vi "Initialize.vi"(8 "error in (no error)":errorcluster, 10 "DeviceName":string, 11 "MagSpec_Bella in":refnum<class "MagSpec_Bella.lvclass">) -> (0 "error out":errorcluster, 1 "new command(s)":string, 2 "DeviceName":string, 3 "MagSpec_Bella out":refnum<class "MagSpec_Bella.lvclass">)   [LabVIEW 2020, in "MagSpec_Bella.lvclass"]
uses:
  MagSpec_Bella.lvclass
  source/Device Drivers/BaseDriver/BaseDriver.lvclass
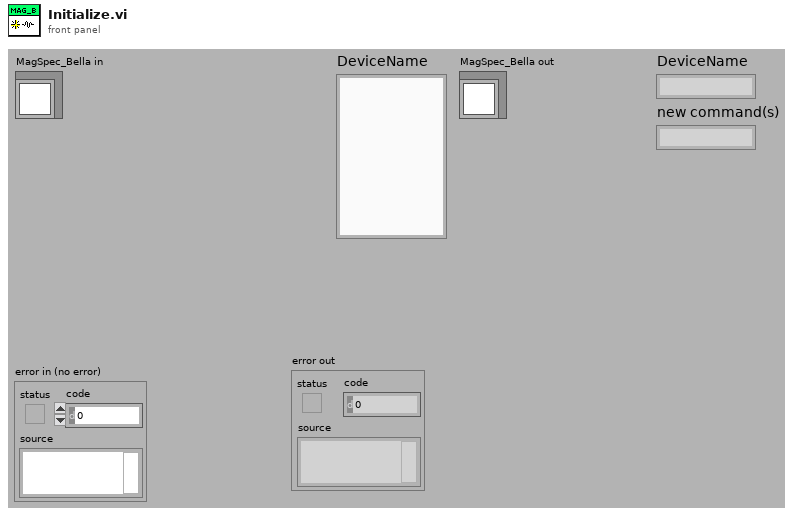
[diagram p1: front panel]
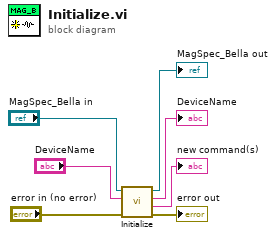
[diagram p0: block diagram]
diagram:
  n1 = call-parent "Initialize.vi"("error in (no error)"="error in (no error)", "DeviceName"="DeviceName", "BaseDriver in"="MagSpec_Bella in") -> ("error out"=→"error out":errorcluster, "new command(s)"=→"new command(s)":string, "DeviceName"=→"DeviceName":string, "BaseDriver out"=→"MagSpec_Bella out":refnum<class "MagSpec_Bella.lvclass">)  [unwired: 5 in]
